vi "RXfilter.vi"(9 "Array":cdb[](array[numeric]), 10 "span":dbl, 11 "sps":dbl) -> (3 "out":cdb[](array[numeric]))   [LabVIEW 2013]
uses:
  <vilib>/imath/engines/lvmath2/RunTimeEngine/ErrorHandling/NIMS_Finalize Error.vi
  <vilib>/imath/engines/lvmath2/RunTimeEngine/NodeEndStatement/NIMS_NodeEndStatement_Output.vi
  <instcachedir>/0/NIMS_NodeEndStatement_Output_53EC0D466D134D7ABD903AC30B43404B.lvgen/NIMS_NodeEndStatement_Output_53EC0D466D134D7ABD903AC30B43404B_000.vi
  LabVIEW Data/MathScriptVIs/MCStatic_31879994332_6309011b735c7d3bdc345e9dbe068425.vi
  <instcachedir>/0/MCStatic_31879994332_6309011b735c7d3bdc345e9dbe068425_26C83AF4E6B94C66802D7F534C05881C.lvgen/MCStatic_31879994332_6309011b735c7d3bdc345e9dbe068425_26C83AF4E6B94C66802D7F534C05881C_000.vi
  MATLAB_func/RX_RRC_filtering.m
  MATLAB_func/rtrcpulse.m
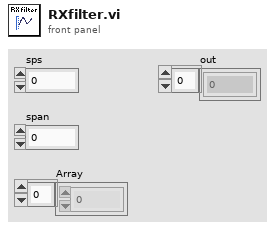
[diagram p1: front panel]
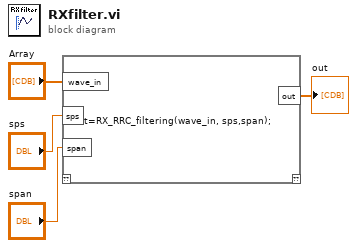
[diagram p0: block diagram]
diagram:
  n1 = mathscript code="out=RX_RRC_filtering(wave_in, sps,span);"("wave_in"="Array", "sps"="sps", "span"="span") -> ("out"=→"out":cdb[])  [unwired: 1 in, 1 out]
